vi "Average trial times for Pump WP.vi"(6 "appended array":dbl[][](array[numeric]), 7 "Photon #":i32=300, 9 "N":i32) -> (0 "At least N values?":bool, 1 "At least 1 value?":bool, 2 "Last WP angle":dbl, 3 "Output":dbl, 4 "Number of values with specified photon #":i16)   [LabVIEW 2013]
panel:
  out "Average (up to N)":dbl
  out "Array":dbl[](array[numeric])
  out "0, 1":i16[](array[numeric])
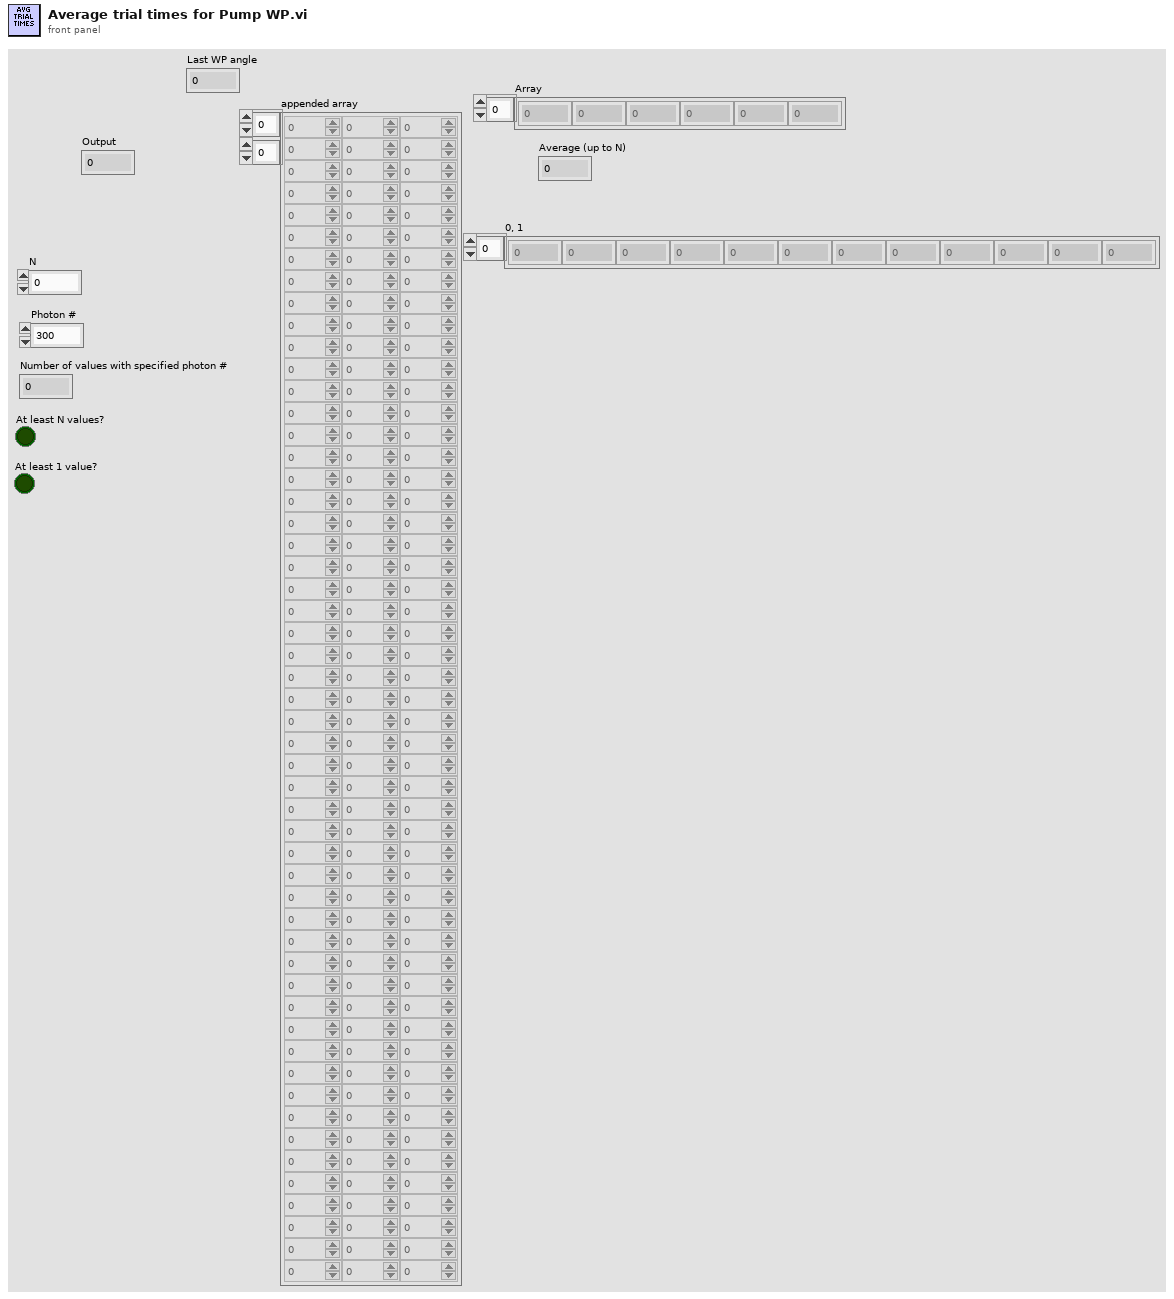
[diagram p1: front panel]
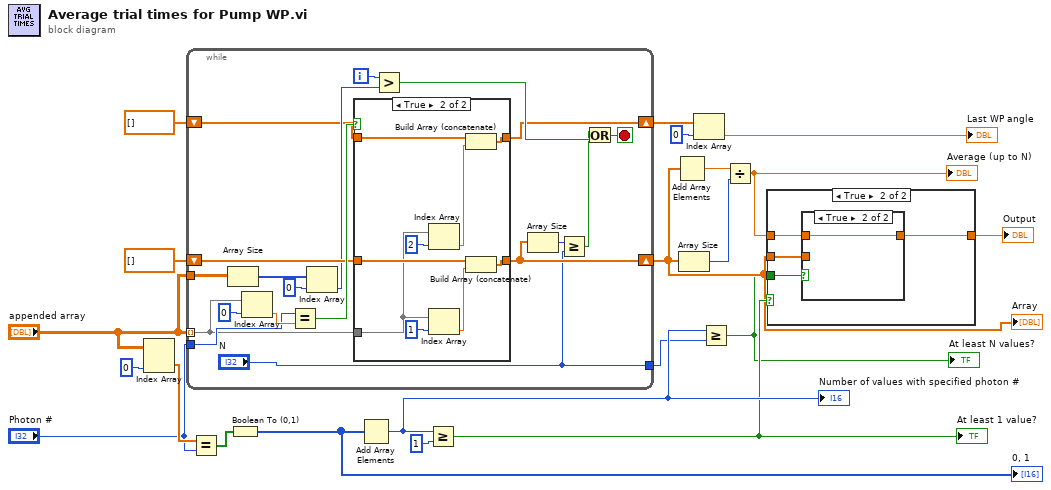
[diagram p0: block diagram]
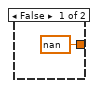
[diagram p2: hidden frame]
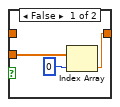
[diagram p3: hidden frame]
diagram:
  n1 = Index Array(array="appended array", index (col)=0 ("disabled index (col)")) -> (element=w18:dbl[])  [unwired: 1 in]
  n2 = while {
    tunnel: "appended array" -> [w36] mode=indexing
    tunnel: "Photon #" -> [w38]
    shift-right: [w34] -> w9
    shift-left: dbl[] [] -> [w35]
    tunnel: "appended array" -> [w32]
    tunnel: ["N"] -> w1
    shift-right: [w22] -> w5
    shift-left: dbl[] [] -> [w23]
    i -> [w31]
    stop <- w25 stop-if-true
    n3 = Array Size(array=w32) -> (size(s)=w30:i32[])
    n4 = Index Array(array=w36, index=0) -> (element=w39:dbl)
    n5 = Equal?(x=w38, y=w39) -> (x = y?=w37:bool)
    n6 = Index Array(array=w30, index=0) -> (element=w28:i32)
    n7 = case shown="True" w37 {
      tunnel: w36 -> [_ w46]
      tunnel: [w42 w49] -> w34
      tunnel: w35 -> [w42 w48]
      tunnel: [w41 w44] -> w22
      tunnel: w23 -> [w41 w43]
      frame False {
      }
      frame True {
        n8 = Index Array(array=w46, index=2) -> (element=w45:dbl)
        n9 = Index Array(array=w46, index=1) -> (element=w50:dbl)
        n10 = Build Array (concatenate)(w43, w45) -> (w44:dbl[])
        n11 = Build Array (concatenate)(w48, w50) -> (w49:dbl[])
      }
    }
    n12 = Greater?(x=w31, y=w28) -> (0:w27:bool)
    n13 = Array Size(array=w34) -> (size(s)=w33:i32)
    n14 = Greater Or Equal?(x=w33, y="N") -> (x >= y?=w26:bool)
    n15 = Or(x=w26, y=w27) -> (x .or. y?=w25:bool)
  }
  "Array" <- w9
  n16 = Equal?(x=w18, y="Photon #") -> (x = y?=w21:bool[])
  n17 = Boolean To (0,1)(Boolean=w21) -> (0, 1=w20:i16[])
  "0, 1" <- w20
  n18 = Add Array Elements(numeric array=w20) -> (sum=w12:i16)
  "Number of values with specified photon #" <- w12
  n19 = Greater Or Equal?(x=w12, y=i16 1) -> (x >= y?=w10:bool)
  "At least 1 value?" <- w10
  n20 = Add Array Elements(numeric array=w9) -> (sum=w14:dbl)
  n21 = Array Size(array=w9) -> (size(s)=w13:i32)
  n22 = Index Array(array=w5, index=0) -> (element=→"Last WP angle":dbl)
  n23 = Greater Or Equal?(x=w12, y=w1) -> (x >= y?=w7:bool)
  "At least N values?" <- w7
  n24 = Divide(x=w14, y=w13) -> (x/y=w6:dbl)
  "Average (up to N)" <- w6
  n25 = case shown="True" w10 {
    tunnel: w9 -> [_ w56]
    tunnel: [nan ("Pump WP") w55] -> w8
    tunnel: w7 -> [_ w54]
    tunnel: w6 -> [_ w53]
    frame False {
    }
    frame True {
      n26 = case shown="True" w54 {
        tunnel: w56 -> [w59 _]
        tunnel: [w57 w60] -> w55
        tunnel: w53 -> [_ w60]
        frame False {
          n27 = Index Array(array=w59, index=0) -> (element=w57:dbl)
        }
        frame True {
        }
      }
    }
  }
  "Output" <- w8
